vi "setTerm.vi"(9 "Height (in)":dbl, 10 "Width (in)":dbl, 11 "String in":string) -> (3 "String out":string, 4 "command":string)   [LabVIEW 2012]
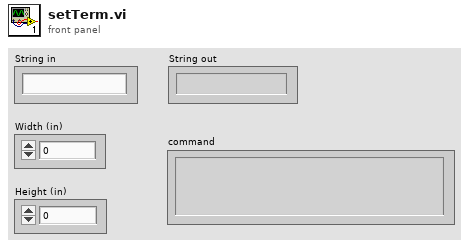
[diagram p1: front panel]
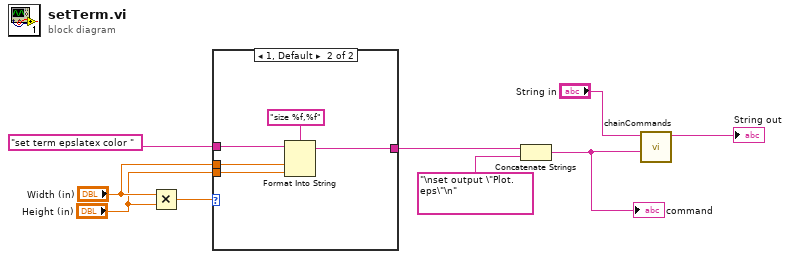
[diagram p0: block diagram]
diagram:
  n1 = Multiply(x="Width (in)", y="Height (in)") -> (x*y=w5:dbl)
  n2 = case shown="1, Default" w5 {
    tunnel: "set term epslatex color " -> [w10 w14]
    tunnel: [w10 w13] -> w8
    tunnel: "Width (in)" -> [_ w12]
    tunnel: "Height (in)" -> [_ w11]
    frame 0 {
    }
    frame 1, Default {
      n3 = Format Into String(format string="size %f,%f", initial string=w14, w12, w11) -> (resulting string=w13:string)  [unwired: 1 in, 1 out]
    }
  }
  n4 = Concatenate Strings(w8, "\nset output \"Plot.eps\"\n") -> (w3:string)
  "command" <- w3
  n5 = call "chainCommands.vi"("Command"=w3, "StringIn"="String in") -> ("StringOut"=→"String out":string)  [unwired: 9 in]
